vi "radar_sample.vi"(4 "error in":errorcluster, 7 "Raw data":string) -> (0 "error out":errorcluster, 3 "Radar Sample":T1)   [LabVIEW 2019, in "Lib_Simx.lvlib"]
doc: "Format the Radar sample into the final format for user display. Include the number of target detected."
uses:
  Lib_Simx.lvlib
  controls/radarSample.ctl
  controls/RadarTrack.ctl
  controls/radar.ctl
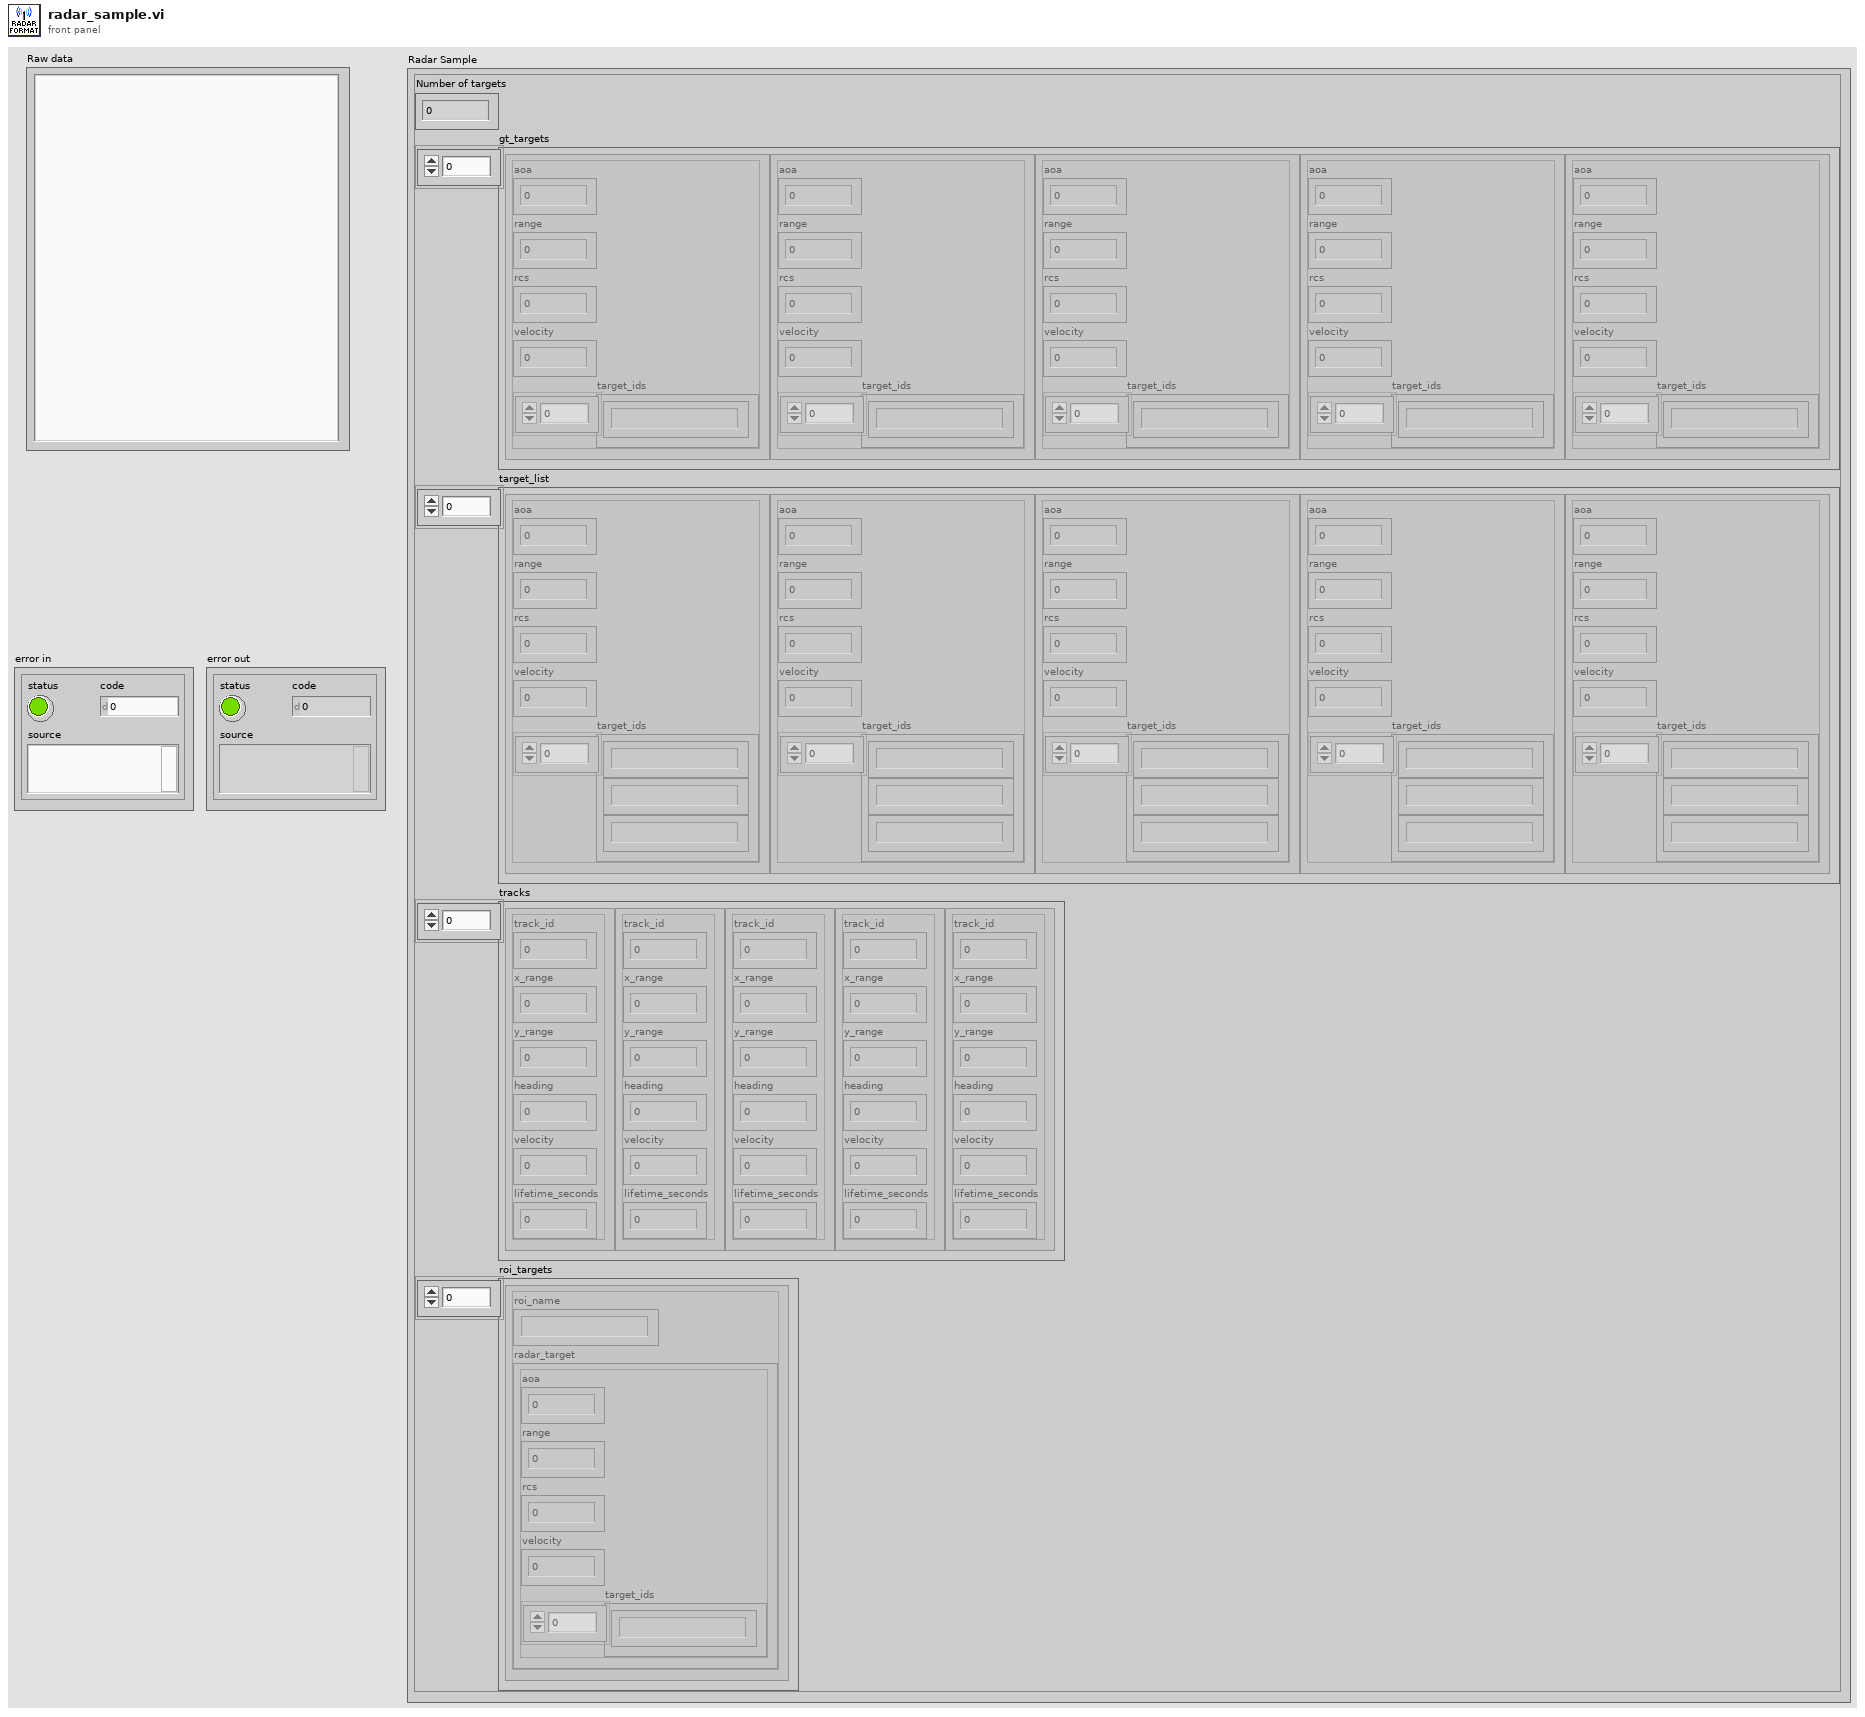
[diagram p1: front panel]
types:
  T1 = typedef "Lib_Simx.lvlib/radarSample.ctl" = cluster{"Number of targets":i32, "gt_targets":cluster{"aoa":sgl, "range":sgl, "rcs":sgl, "velocity":sgl, "target_ids":string[]}[], "target_list":cluster{"aoa":sgl, "range":sgl, "rcs":sgl, "velocity":sgl, "target_ids":string[]}[], "tracks":T2[], "roi_targets":cluster{"roi_name":string, "radar_target":cluster{"aoa":sgl, "range":sgl, "rcs":sgl, "velocity":sgl, "target_ids":string[]}}[]}
  T2 = typedef "Lib_Simx.lvlib/RadarTrack.ctl" = cluster{"track_id":u64, "x_range":sgl, "y_range":sgl, "heading":sgl, "velocity":sgl, "lifetime_seconds":sgl}
  T3 = typedef "Lib_Simx.lvlib/radar.ctl" = cluster{"gt_targets":cluster{"aoa":sgl, "range":sgl, "rcs":sgl, "velocity":sgl, "target_ids":string[]}[], "target_list":cluster{"aoa":sgl, "range":sgl, "rcs":sgl, "velocity":sgl, "target_ids":string[]}[], "tracks":T2[], "roi_targets":cluster{"roi_name":string, "radar_target":cluster{"aoa":sgl, "range":sgl, "rcs":sgl, "velocity":sgl, "target_ids":string[]}}[]}
  T4 = cluster{"aoa":sgl, "range":sgl, "rcs":sgl, "velocity":sgl, "target_ids":string[]}[]
  T5 = cluster{"roi_name":string, "radar_target":cluster{"aoa":sgl, "range":sgl, "rcs":sgl, "velocity":sgl, "target_ids":string[]}}[]
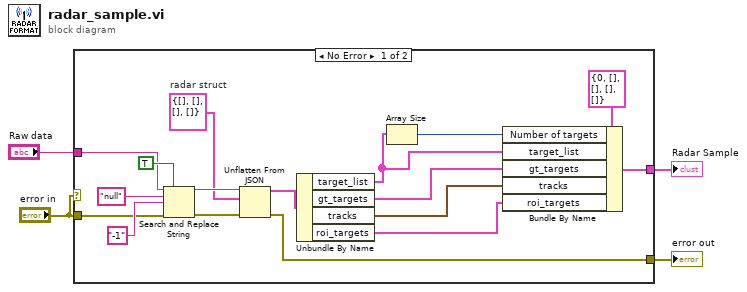
[diagram p0: block diagram]
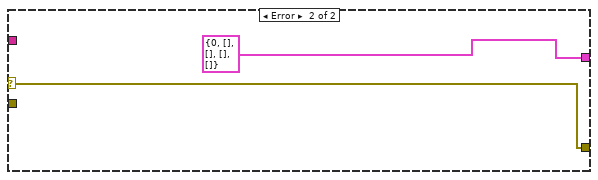
[diagram p2: hidden frame]
diagram:
  n1 = case shown="No Error" "error in" {
    selector: "error in" -> [_ w22]
    tunnel: [w21 T1 {"Number of targets"=0, "gt_targets"=[], "target_list"=[], "tracks"=[], "roi_targets"=[]} ("Radar 2")] -> w4
    tunnel: [w15 w22] -> w3
    tunnel: "error in" -> [w8 _]
    tunnel: "Raw data" -> [w9 _]
    frame No Error {
      w5 = T3 {"gt_targets"=[], "target_list"=[], "tracks"=[], "roi_targets"=[]}  # radar struct
      n2 = Search and Replace String(replace all?=TRUE ("replace all? (F)"), input string=w9, search string="null", replace string="-1" ("replace string (\"\")"), error in=w8) -> (result string=w6:string, error out=w7:errorcluster)  [unwired: 3 in, 2 out]
      n3 = Unflatten From JSON(JSON string=w6, type and defaults=w5, error in (no error)=w7) -> (value=w16:T3, error out=w15:errorcluster)  [unwired: 4 in]
      n4 = Unbundle By Name(w16) -> ("target_list"=w18:T4, "gt_targets"=w19:T4, "tracks"=w14:T2[], "roi_targets"=w13:T5)
      n5 = Array Size(array=w18) -> (size(s)=w17:i32)
      n6 = Bundle By Name(cluster=T1 {"Number of targets"=0, "gt_targets"=[], "target_list"=[], "tracks"=[], "roi_targets"=[]} ("Radar 2"), "Number of targets"=w17, "target_list"=w18, "gt_targets"=w19, "tracks"=w14, "roi_targets"=w13) -> (w21:T1)
    }
    frame Error {
    }
  }
  "Radar Sample" <- w4
  "error out" <- w3
